vi "FTW-Expression-Destroy.vi"(0 "Expression":refnum<class "FTW-Expression.lvclass">, 11 "error in":errorcluster) -> (15 "error out":errorcluster)   [LabVIEW 2015, in "FTW-Expression.lvclass"]
uses:
  FTW-Expression.lvclass
  FTW-Expression.lvclass/FTW-Expression.ctl
panel:
  # "Inputs"
  # "Outputs"
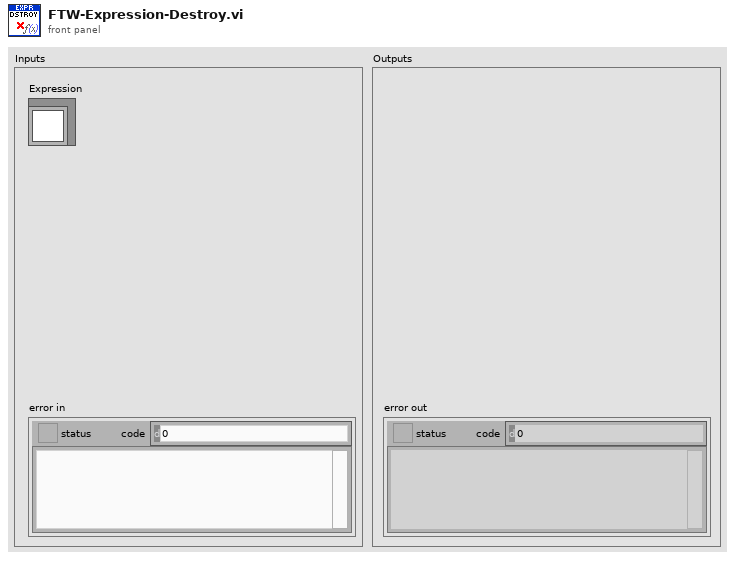
[diagram p1: front panel]
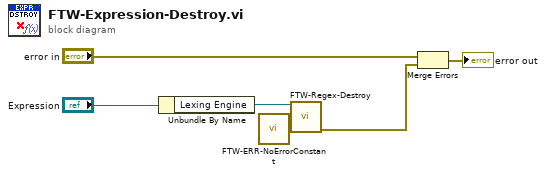
[diagram p0: block diagram]
diagram:
  n1 = Unbundle By Name("Expression") -> ("Lexing Engine"=w2:refnum<data-value>)
  n2 = call "FTW-ERR-NoErrorConstant.vi"() -> ("no error"=w3:errorcluster)
  n3 = call "FTW-Regex-Destroy.vi"("Regex"=w2, "error in"=w3) -> ("error out"=w1:errorcluster)  [unwired: 13 in]
  n4 = Merge Errors("error in", w1) -> (→"error out":errorcluster)
